vi "CM-Select Slot Controls.vi"(0 "slot ctl refs":refnum<vi>[](array[refnum]), 5 "Devices":T1[](array[typedef]), 9 "Breakout box type":enum32{"BNC-2090", "BNC-2110"}(radio), 11 "error in (no error)":errorcluster) -> (4 "slot ctl refs out":refnum<vi>[](array[refnum]), 6 "Devices thru":T1[](array[typedef]), 15 "error out":errorcluster)   [LabVIEW 2015]
uses:
  Type Defs/General PXISlot XControl/PXISlotGP.xctl
  PXI DAQ VIs/Type Defs/PXI-Device Spec.ctl
  Type Defs/PXISlot XControl/Connector Type.ctl
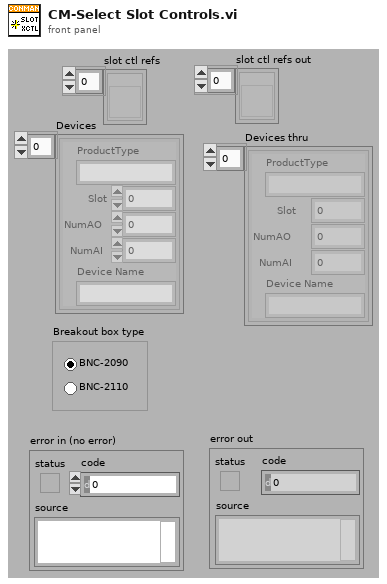
[diagram p1: front panel]
types:
  T1 = typedef "PXI-Device Spec.ctl" = cluster{"Slot":i32, "ProductType":string, "NumAO":i32, "NumAI":i32, "Device Name":string}
  T2 = typedef "Connector Type.ctl" = enum16{"None", "PXI-4461", "BNC-2110", "BNC-2090"}
  T3 = cluster{"Output sources":string[], "Input sources":string[]}
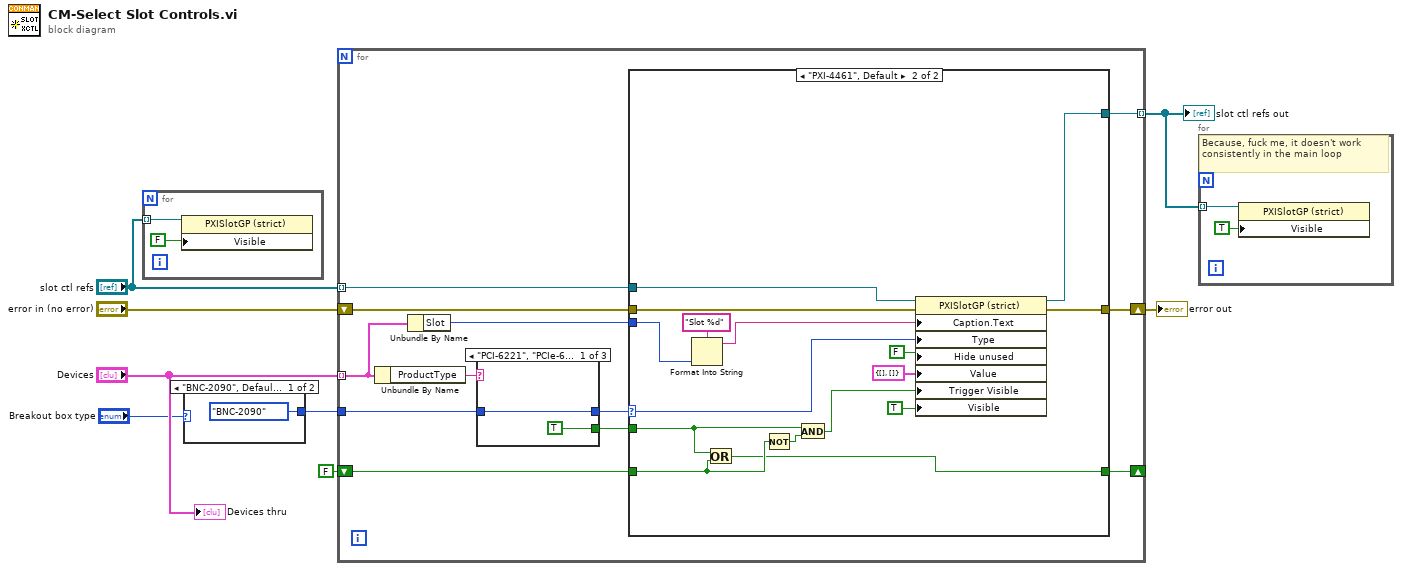
[diagram p0: block diagram]
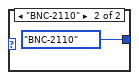
[diagram p2: hidden frame]
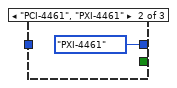
[diagram p3: hidden frame]
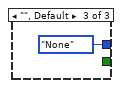
[diagram p4: hidden frame]
diagram:
  n1 = for {
    tunnel: "slot ctl refs" -> [w10] mode=indexing
    n2 = property class="PXISlotGP (strict)"(reference=w10, "Visible"=FALSE) -> ()  [unwired: 1 in, 2 out]
  }
  n3 = case shown="\"BNC-2090\", Default" "Breakout box type" {
    tunnel: [Connector_Type."BNC-2090" ("Connector Type") Connector_Type."BNC-2110" ("Connector Type")] -> w1
    frame "BNC-2090", Default {
    }
    frame "BNC-2110" {
    }
  }
  n4 = for {
    tunnel: "slot ctl refs" -> [w22] mode=indexing
    shift-right: [w23] -> w7
    shift-left: "error in (no error)" -> [w24]
    tunnel: "Devices" -> [w17] mode=indexing
    tunnel: w1 -> [w20]
    shift-right: [w15] -> _
    shift-left: FALSE -> [w16]
    tunnel: [w13] -> w5 mode=indexing
    n5 = Unbundle By Name(w17) -> ("ProductType"=w21:string)
    n6 = Unbundle By Name(w17) -> ("Slot"=w14:i32)
    n7 = case shown="\"PCI-6221\", \"PCIe-6321\", \"PXI-6221\", \"PXIe-6341\", \"USB-6002\", \"USB-6221 (BNC)\", \"USB-6341 (BNC)\"" w21 {
      tunnel: w20 -> [w26 _ _]
      tunnel: [w26 Connector_Type."PXI-4461" ("Connector Type") Connector_Type."None" ("Connector Type")] -> w19
      tunnel: [TRUE _ _] -> w18
      frame "PCI-6221", "PCIe-6321", "PXI-6221", "PXIe-6341", "USB-6002", "USB-6221 (BNC)", "USB-6341 (BNC)" {
      }
      frame "PCI-4461", "PXI-4461" {
      }
      frame "", Default {
      }
    }
    n8 = case shown="\"PXI-4461\", Default" w19 {
      selector: w19 -> [_ w42]
      tunnel: w24 -> [w30 w46]
      tunnel: [w30 w45] -> w23
      tunnel: w22 -> [_ w34]
      tunnel: [_ w35] -> w13
      tunnel: w14 -> [_ w32]
      tunnel: w18 -> [_ w38]
      tunnel: w16 -> [w29 w37]
      tunnel: [w29 w36] -> w15
      frame "None" {
      }
      frame "PXI-4461", Default {
        n9 = Format Into String(format string="Slot %d", w32) -> (resulting string=w31:string)  [unwired: 2 in, 1 out]
        n10 = Or(x=w38, y=w37) -> (x .or. y?=w36:bool)
        n11 = Not(x=w37) -> (.not. x?=w40:bool)
        n12 = And(x=w38, y=w40) -> (x .and. y?=w39:bool)
        n13 = property class="PXISlotGP (strict)"(reference=w34, error in=w46, "Caption.Text"=w31, "Type"=w42, "Hide unused"=FALSE, "Value"=T3 {"Output sources"=[], "Input sources"=[]}, "Trigger Visible"=w39, "Visible"=TRUE) -> (reference out=w35:refnum<vi>, error out=w45:errorcluster)
      }
    }
  }
  "error out" <- w7
  "slot ctl refs out" <- w5
  n14 = for {
    tunnel: w5 -> [w48] mode=indexing
    # "Because, fuck me, it doesn't work consistently in the main loop"
    n15 = property class="PXISlotGP (strict)"(reference=w48, "Visible"=TRUE) -> ()  [unwired: 1 in, 2 out]
  }
  "Devices thru" <- "Devices"
